vi "Set View by Tab Index.vi"(8 "error in (no error)":errorcluster, 10 "Index":i32, 11 "TabbedViewManager In":refnum<class "TabbedViewManager.lvclass">) -> (0 "error out":errorcluster, 3 "TabbedViewManager Out":refnum<class "TabbedViewManager.lvclass">)   [LabVIEW 2015, in "TabbedViewManager.lvlib" / "TabbedViewManager.lvclass"]
doc: "<License>\nCopyright © 2017 Composed Systems, LLC | All rights reserved\nwww.composed.io\n\nAuthor: Ethan Stern <ethan.stern@composed.io>\n\nThis software is provided \"AS IS\" WITHOUT WARRANTIES, either express or implied, AND IS FOR EDUCATIONAL PURPOSES ONLY.\n</License>"
uses:
  TabbedViewManager.lvclass
  Framework/IViewManager/IViewManager/IViewManager.lvclass/IViewManager.ctl
  TabbedViewManager.lvclass/TabbedViewManager.ctl
  Framework/IViewable/IViewable Messages/Insert Front Panel Msg/Insert Front Panel Msg.lvclass/Insert Front Panel Msg.ctl
  <vilib>/ActorFramework/Message Enqueuer/Message Enqueuer.lvclass/Message Enqueuer.ctl
  <vilib>/ActorFramework/Message Enqueuer/Enqueue.vi
  <vilib>/ActorFramework/Message Priority Queue/Priority Enqueue.vi
  Framework/IViewable/IViewable Messages/Insert Front Panel Msg/Insert Front Panel Msg.lvclass
  Framework/IViewManager/IViewManager/IViewManager.lvclass
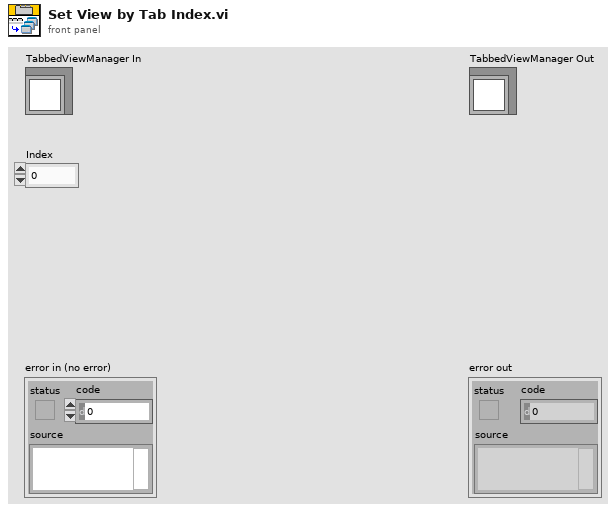
[diagram p1: front panel]
types:
  T1 = typedef "IViewable.lvlib/ProtectedSubpanel.lvclass/Protected Subpanel Reference.ctl" = refnum<data-value>
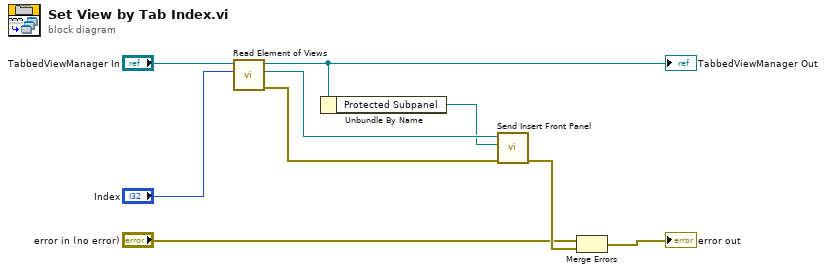
[diagram p0: block diagram]
diagram:
  n1 = call "Read Element of Views.vi"("Index"="Index", "IViewManager In"="TabbedViewManager In") -> ("error out"=w5:errorcluster, "View Ref"=w6:refnum<class "Message Enqueuer.lvclass">, "IViewManager Out"=w7:refnum<class "TabbedViewManager.lvclass">)  [unwired: 7 in]
  "TabbedViewManager Out" <- w7
  n2 = Unbundle By Name(w7) -> ("Protected Subpanel"=w4:T1)
  n3 = call "Send Insert Front Panel.vi"("error in (no error)"=w5, "Protected Subpanel"=w4, "Message Enqueuer"=w6) -> ("error out"=w9:errorcluster)  [unwired: 7 in, 1 out]
  n4 = Merge Errors("error in (no error)", w9) -> (→"error out":errorcluster)
